vi "(SubVI)I2C_Wait until Check the Register.vi"(4 "Delay (10)":u32=10, 5 "Log Ref":refnum<vi>, 6 "Loop Count (50)":i32=50, 8 "error in (no error)":errorcluster caption="에러 입력(에러 없음)", 9 "Ref Data":u16 format="%04x", 10 "Address":u16 format="%04x", 11 "Slave ID":u8 format="%.0x") -> (0 "error out":errorcluster caption="에러 출력", 1 "Read Data":u16, 2 "Log":string, 3 "Pass?":bool)   [LabVIEW 2020]
uses:
  Instance VIs/(SubVI)I2C_16Bit-16Bit_Read_Single.vi
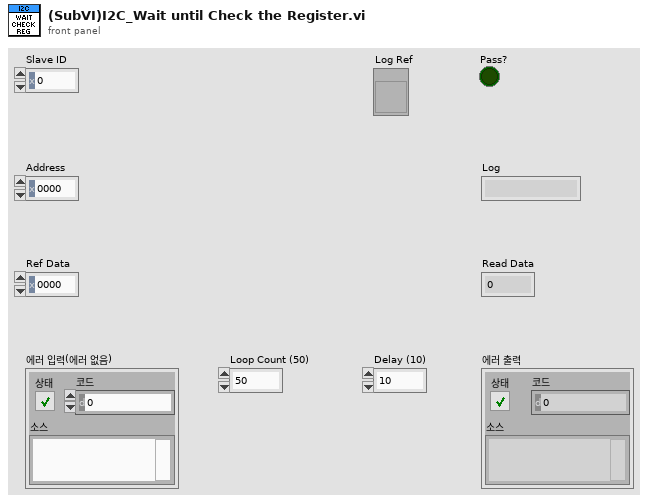
[diagram p1: front panel]
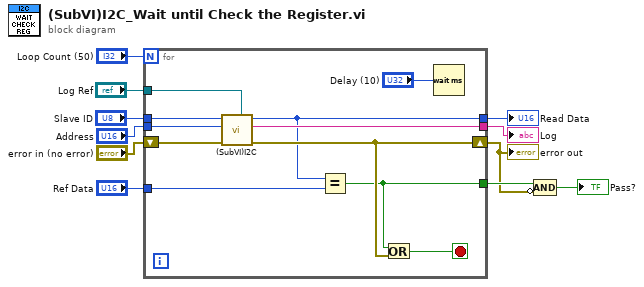
[diagram p0: block diagram]
diagram:
  n1 = for {
    N: "Loop Count (50)" -> [_]
    tunnel: "Slave ID" -> [w21]
    tunnel: "Address" -> [w20]
    tunnel: "Ref Data" -> [w19]
    shift-right: [w16] -> w2
    shift-left: "error in (no error)" -> [w17]
    tunnel: "Log Ref" -> [w15]
    tunnel: [w14] -> w3
    tunnel: [w13] -> w6
    tunnel: [w12] -> w4
    stop <- w18 stop-if-true
    n2 = call-poly "(SubVI)I2C.vi"("Log Ref"=w15, "error in (no error)"=w17, "Address"=w20, "ID"=w21) -> ("error out"=w16:errorcluster, "Log"=w13:string, "Read Data"=w12:u16)  [unwired: 5 in]
    n3 = Equal?(x=w12, y=w19) -> (x = y?=w14:bool)
    n4 = Or(x=w14, y=w16) -> (x .or. y?=w18:bool)
    n5 = Wait (ms)(milliseconds to wait="Delay (10)") -> ()  [unwired: 1 out]
  }
  "error out" <- w2
  "Log" <- w6
  "Read Data" <- w4
  n6 = Compound Arithmetic op=AND(w3, invert w2) -> (→"Pass?":bool)
